vi "nelder_evaluate_shrink.vi"(8 "error in":errorcluster, 9 "settling time":u32, 10 "shrink point":sgl[][](array[numeric]), 11 "Cluster":T2) -> (0 "error out":errorcluster, 2 "f_val2":dbl, 3 "f_val1":dbl)   [LabVIEW 2018]
uses:
  C:/Program Files/National Instruments/LabVIEW 2018/instr.lib/IDS/ueye.NET/uEyeDotNet.dll
  <userlib>/PDamp/PDref.ctl
  <userlib>/PDamp/channel.ctl
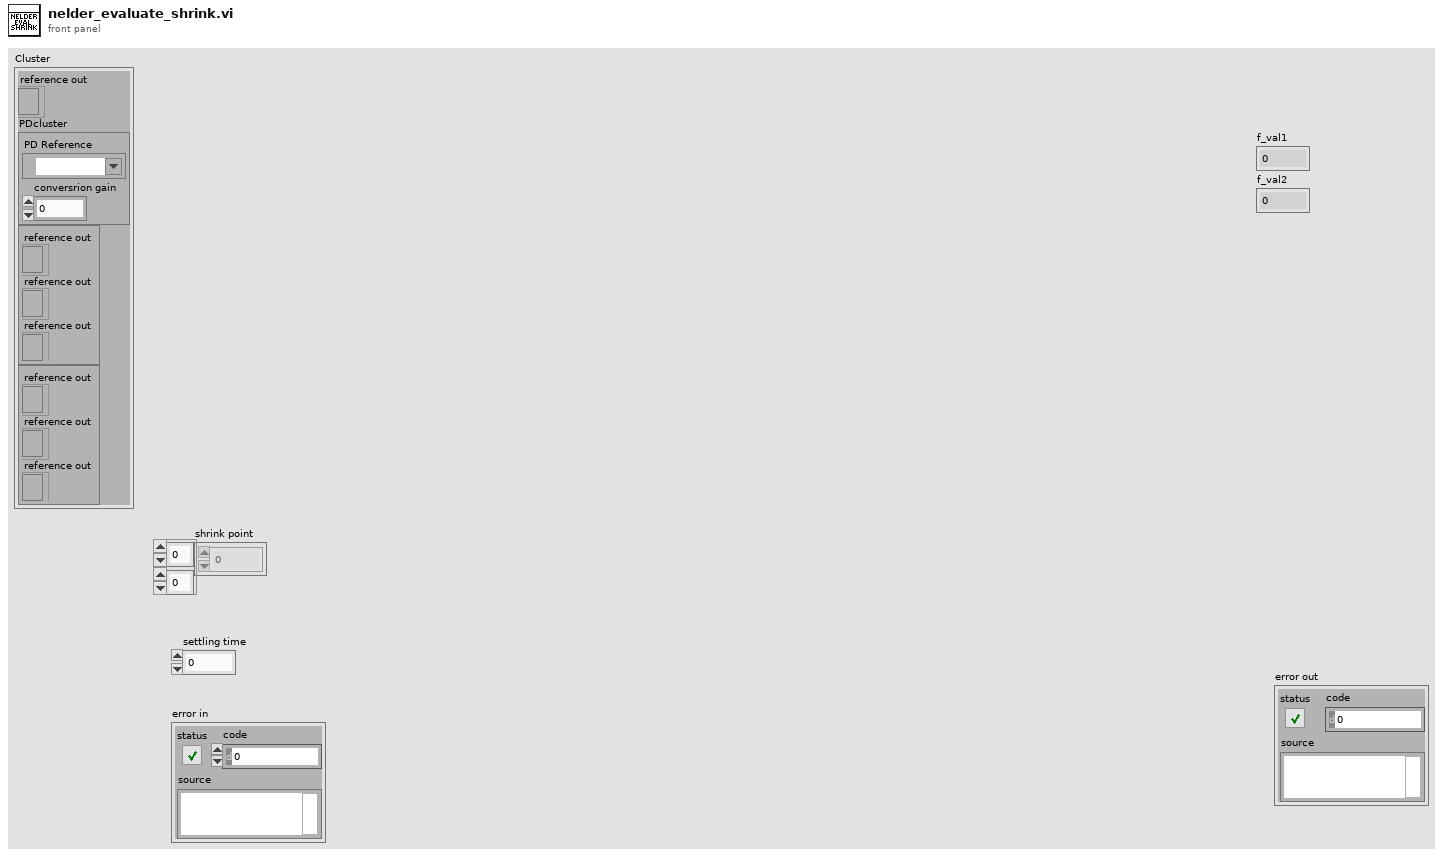
[diagram p1: front panel]
types:
  T1 = typedef "PDref.ctl" = cluster{"PD Reference":refnum<visa-resource-name>, "conversrion gain":dbl}
  T2 = cluster{"reference out":refnum<k24>, "PDcluster":T1, cluster{"reference out":refnum<k7>, "reference out":refnum<k7>, "reference out":refnum<k7>}, cluster{"reference out":refnum<k7>, "reference out":refnum<k7>, "reference out":refnum<k7>}}
  T3 = cluster{"reference out":refnum<k7>, "reference out":refnum<k7>, "reference out":refnum<k7>}
  T4 = typedef "channel.ctl" = enum16{"ch1", "ch2", "ch3", "ch4"}
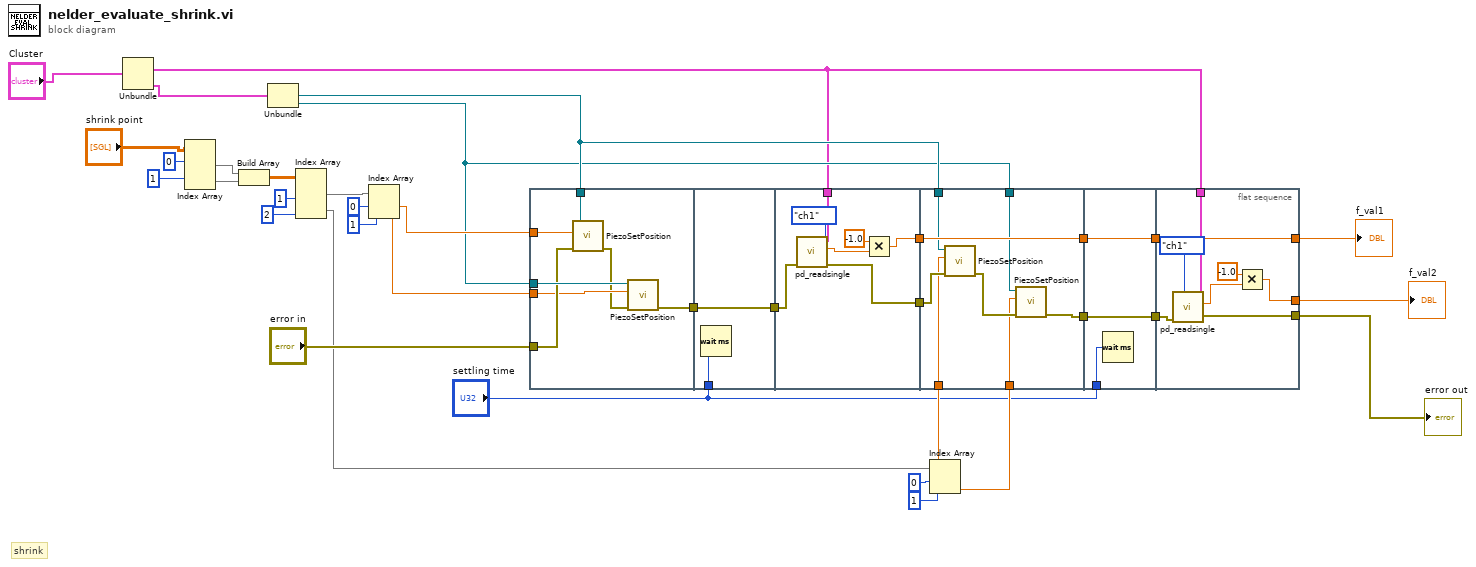
[diagram p0: block diagram]
diagram:
  # "shrink"
  n1 = Unbundle("Cluster") -> ("PDcluster"=w7:T1, w34:T3)  [unwired: 2 out]
  n2 = Index Array(array="shrink point", index (row) #1=0 ("index (row)"), index (row) #2=1 ("index (row)")) -> (element #1=w29:sgl[], element #2=w30:sgl[])  [unwired: 2 in]
  n3 = Build Array(w29, w30) -> (w28:sgl[][])
  n4 = Unbundle(w34) -> ("reference out"=w19:refnum<k7>, "reference out"=w13:refnum<k7>)  [unwired: 1 out]
  n5 = Index Array(array=w28, index (col) #1=1 ("disabled index (col)"), index (col) #2=2 ("index (col)")) -> (element #1=w24:sgl[], element #2=w16:sgl[])  [unwired: 2 in]
  n6 = Index Array(array=w24, index #1=0 ("index"), index #2=1 ("index")) -> (element #1=w21:sgl, element #2=w20:sgl)
  n7 = flat-sequence {
    tunnel: w19 -> [w43]
    tunnel: w13 -> [w42]
    tunnel: [w37] -> w36
    tunnel: "error in" -> [w41]
    tunnel: w21 -> [w40]
    tunnel: w20 -> [w39]
    tunnel: "settling time" -> [w45]
    tunnel: [w44] -> w35
    tunnel: w36 -> [w44]
    tunnel: w7 -> [w52]
    tunnel: w35 -> [w50]
    tunnel: [w46] -> w12
    tunnel: [w49] -> w11
    tunnel: w12 -> [w60]
    tunnel: w11 -> [w59]
    tunnel: w19 -> [w57]
    tunnel: w15 -> [w56]
    tunnel: w14 -> [w55]
    tunnel: w13 -> [w54]
    tunnel: [w60] -> w10
    tunnel: [w53] -> w6
    tunnel: w10 -> [w63]
    tunnel: "settling time" -> [w62]
    tunnel: [w63] -> w8
    tunnel: w6 -> [w61]
    tunnel: [w61] -> w5
    tunnel: [w71] -> w3
    tunnel: w8 -> [w71]
    tunnel: w7 -> [w70]
    tunnel: w5 -> [w69]
    tunnel: [w64] -> w2
    tunnel: [w67] -> w4
    frame #0 {
      n8 = call <userlib>:"PiezoSetPosition.vi"("error in (no error)"=w41, "pos in"=w40, "reference"=w43) -> ("error out"=w38:errorcluster)  [unwired: 3 in, 1 out]
      n9 = call <userlib>:"PiezoSetPosition.vi"("error in (no error)"=w38, "pos in"=w39, "reference"=w42) -> ("error out"=w37:errorcluster)  [unwired: 3 in, 1 out]
    }
    frame #1 {
      n10 = Wait (ms)(milliseconds to wait=w45) -> ()  [unwired: 1 out]
    }
    frame #2 {
      n11 = call <userlib>:"pd_readsingle.vi"("PDcluster in"=w52, "channel"=channel."ch1", "error in (no error)"=w50) -> ("photocurrent"=w47:dbl, "error out"=w49:errorcluster)  [unwired: 5 in, 1 out]
      n12 = Multiply(x=-1.0, y=w47) -> (x*y=w46:dbl)
    }
    frame #3 {
      n13 = call <userlib>:"PiezoSetPosition.vi"("error in (no error)"=w59, "pos in"=w56, "reference"=w57) -> ("error out"=w58:errorcluster)  [unwired: 3 in, 1 out]
      n14 = call <userlib>:"PiezoSetPosition.vi"("error in (no error)"=w58, "pos in"=w55, "reference"=w54) -> ("error out"=w53:errorcluster)  [unwired: 3 in, 1 out]
    }
    frame #4 {
      n15 = Wait (ms)(milliseconds to wait=w62) -> ()  [unwired: 1 out]
    }
    frame #5 {
      n16 = call <userlib>:"pd_readsingle.vi"("PDcluster in"=w70, "channel"=channel."ch1", "error in (no error)"=w69) -> ("photocurrent"=w65:dbl, "error out"=w67:errorcluster)  [unwired: 5 in, 1 out]
      n17 = Multiply(x=-1.0, y=w65) -> (x*y=w64:dbl)
    }
  }
  n18 = Index Array(array=w16, index #1=0 ("index"), index #2=1 ("index")) -> (element #1=w15:sgl, element #2=w14:sgl)
  "error out" <- w4
  "f_val1" <- w3
  "f_val2" <- w2
